vi "Actor Core.vi"(8 "error in (no error)":errorcluster, 11 "ADM AF.lvlib:ADM AF.lvclass":refnum<class "ADM AF.lvclass">) -> (0 "error out":errorcluster, 3 "Actor out":refnum<class "Actor.lvclass">)   [LabVIEW 2018, in "ADM AF.lvlib" / "ADM AF.lvclass"]
doc: "This is Actor Core.vi, the main message handling loop for Actors. An actor usually just sits in this loop and processes messages as they arrive. Any error returned by the message Do.vi call will stop the loop, with error code 43 as the canonical signal to stop with no error sent to caller. Descendants may override that in Handle Error.vi."
uses:
  ADM AF.lvclass
  C:/Program Files (x86)/National Instruments/LabVIEW 2018/vi.lib/ActorFramework/Actor/Actor.lvclass
  <vilib>/ActorFramework/Actor/Actor.lvclass
  Stage/Stage.lvclass
  Feeder/Feeder.lvclass
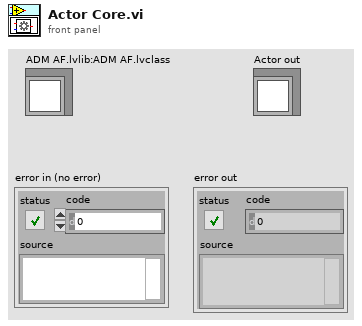
[diagram p1: front panel]
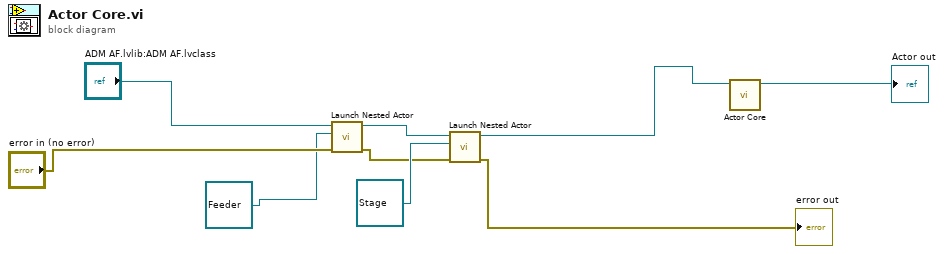
[diagram p0: block diagram]
diagram:
  n1 = call <vilib>:"Launch Nested Actor.vi"("error in (no error)"="error in (no error)", "Nested Actor"=refnum<class "Feeder.lvclass"> refnum ("ADM AF.lvlib:Feeder.lvclass"), "Caller Actor in"="ADM AF.lvlib:ADM AF.lvclass") -> ("error out"=w5:errorcluster, "Caller Actor out"=w9:refnum<class "ADM AF.lvclass">)  [unwired: 6 in, 1 out]
  n2 = call <vilib>:"Launch Nested Actor.vi"("error in (no error)"=w5, "Nested Actor"=refnum<class "Stage.lvclass"> refnum ("ADM AF.lvlib:Stage.lvclass"), "Caller Actor in"=w9) -> ("error out"=→"error out":errorcluster, "Caller Actor out"=w3:refnum<class "ADM AF.lvclass">)  [unwired: 6 in, 1 out]
  n3 = call-parent "Actor Core.vi"("Actor in"=w3) -> ("Actor out"=→"Actor out":refnum<class "Actor.lvclass">)  [unwired: 9 in, 1 out]
